vi "Calculate number of trigger pulses.vi"(8 "error in (no error)":errorcluster, 11 "DAQOrcaFlash in":refnum<class "DAQOrcaFlash.lvclass">) -> (0 "error out":errorcluster, 3 "DAQOrcaFlash out":refnum<class "DAQOrcaFlash.lvclass">)   [LabVIEW 2012, in "DAQOrcaFlash.lvclass"]
uses:
  DAQOrcaFlash.lvclass
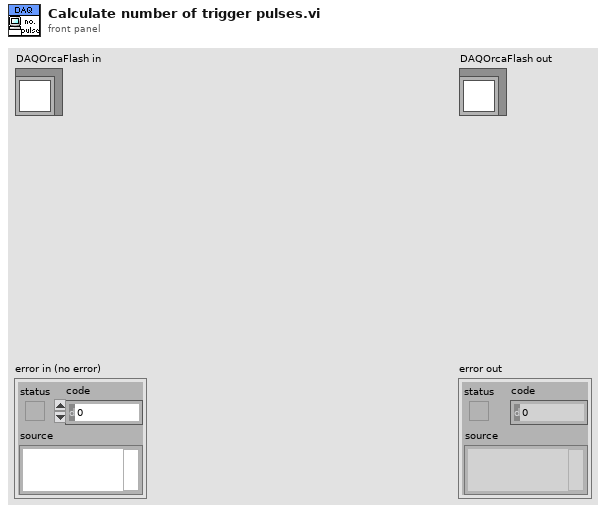
[diagram p1: front panel]
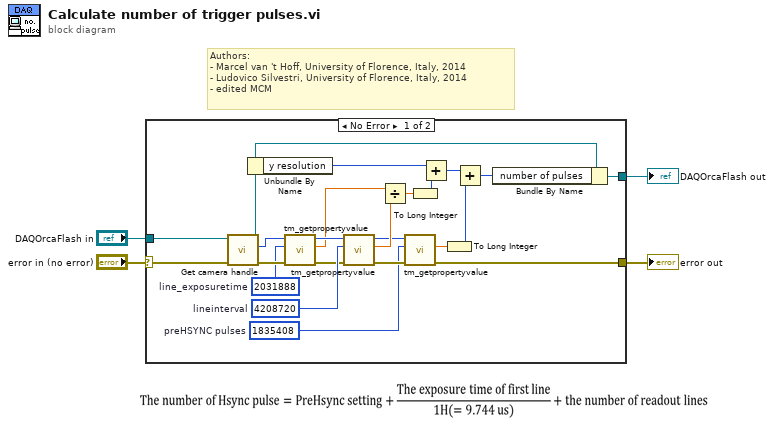
[diagram p0: block diagram]
diagram:
  # "Authors: \n- Marcel van 't Hoff, University of Florence, Italy, 2014\n- Ludovico Silvestri, University of Florence, Italy, 2014\n- edited MCM"
  n1 = case shown="No Error" "error in (no error)" {
    selector: "error in (no error)" -> [w26 w29]
    tunnel: [w10 w29] -> w3
    tunnel: [w27 w28] -> w1
    tunnel: "DAQOrcaFlash in" -> [w24 w28]
    frame No Error {
      w9 = u32 1835408  # preHSYNC pulses
      w19 = u32 2031888  # line_exposuretime
      w22 = u32 4208720  # lineinterval
      n2 = call "Get camera handle.vi"("error in (no error)"=w26, "DAQMH121119OrcaFlash in"=w24) -> ("error out"=w25:errorcluster, "cam handle"=w13:u32, "DAQMH121119OrcaFlash out"=w23:refnum<class "DAQOrcaFlash.lvclass">)  [unwired: 7 in]
      n3 = Unbundle By Name(w23) -> ("y resolution"=w15:i32)
      n4 = call <userlib>:"tm_getpropertyvalue.vi"("error in (no error)"=w25, "Property ID"=w19, "Handle in"=w13) -> ("error out"=w20:errorcluster, "Value in"=w18:sgl, "Handle out"=w21:u32)  [unwired: 6 in]
      n5 = call <userlib>:"tm_getpropertyvalue.vi"("error in (no error)"=w20, "Property ID"=w22, "Handle in"=w21) -> ("error out"=w11:errorcluster, "Value in"=w17:sgl, "Handle out"=w12:u32)  [unwired: 6 in]
      n6 = Divide(x=w18, y=w17) -> (x/y=w16:sgl)
      n7 = call <userlib>:"tm_getpropertyvalue.vi"("error in (no error)"=w11, "Property ID"=w9, "Handle in"=w12) -> ("error out"=w10:errorcluster, "Value in"=w8:sgl)  [unwired: 6 in, 1 out]
      n8 = To Long Integer(number=w16) -> (32bit integer=w14:i32)
      n9 = Add(x=w15, y=w14) -> (x+y=w6:i32)
      n10 = To Long Integer(number=w8) -> (32bit integer=w7:i32)
      n11 = Add(x=w6, y=w7) -> (x+y=w5:i32)
      n12 = Bundle By Name(cluster=w23, "number of pulses"=w5) -> (w27:refnum<class "DAQOrcaFlash.lvclass">)
    }
    frame Error {
    }
  }
  "error out" <- w3
  "DAQOrcaFlash out" <- w1
